vi "Set Frequency.vi"(8 "error in (no error)":errorcluster, 10 "Frequency":dbl format="%#_6pHz", 11 "Lock-in in":refnum<class "Lock-in.lvclass">) -> (0 "error out":errorcluster, 3 "Lock-in out":refnum<class "Lock-in.lvclass">)   [LabVIEW 2016, in "Lock-in.lvclass"]
uses:
  Lock-in.lvclass
  NHMFL_Core/Libraries/Instruments/Instrument Driver/Lock-in Driver/Lock-in Driver.lvclass
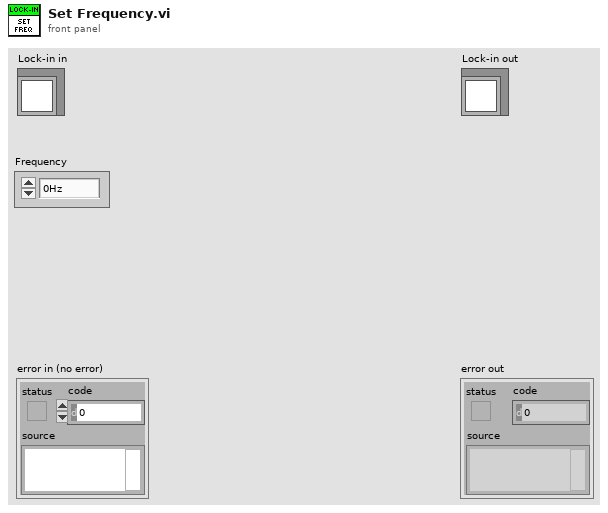
[diagram p1: front panel]
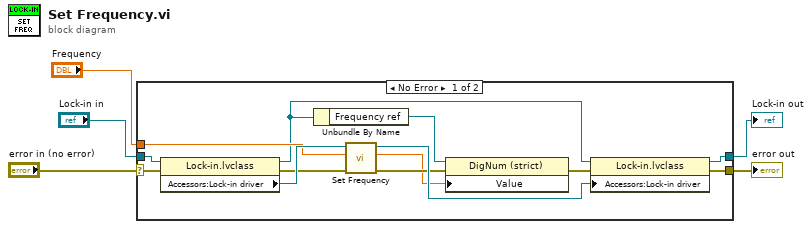
[diagram p0: block diagram]
diagram:
  n1 = case shown="No Error" "error in (no error)" {
    selector: "error in (no error)" -> [w17 w20]
    tunnel: [w11 w20] -> w4
    tunnel: [w12 w19] -> w2
    tunnel: "Lock-in in" -> [w18 w19]
    tunnel: "Frequency" -> [w15 _]
    frame No Error {
      n2 = property class="Lock-in.lvclass"(reference=w18, error in=w17) -> (reference out=w8:refnum<class "Lock-in.lvclass">, error out=w14:errorcluster, "Accessors:Lock-in driver"=w16:refnum<class "Lock-in Driver.lvclass">)
      n3 = Unbundle By Name(w8) -> ("Frequency ref"=w7:refnum<vi>)
      n4 = call-dynamic "Set Frequency.vi"("error in (no error)"=w14, "Frequency"=w15, "Lock-in Driver in"=w16) -> ("error out"=w10:errorcluster, "Actual frequency"=w6:dbl, "Lock-in Driver out"=w13:refnum<class "Lock-in Driver.lvclass">)  [unwired: 6 in]
      n5 = property class="DigNum (strict)"(reference=w7, error in=w10, "Value"=w6) -> (error out=w9:errorcluster)  [unwired: 1 out]
      n6 = property class="Lock-in.lvclass"(reference=w8, error in=w9, "Accessors:Lock-in driver"=w13) -> (reference out=w12:refnum<class "Lock-in.lvclass">, error out=w11:errorcluster)
    }
    frame Error {
    }
  }
  "error out" <- w4
  "Lock-in out" <- w2
